vi "SpinningBooms.vi"() -> ()   [LabVIEW 2016]
doc: "The myRIO Project template acquires acceleration data from the onboard accelerometer and displays the changes of acceleration values in a waveform chart."
uses:
  <vilib>/myRIO/Common/Instrument Driver Framework/myRIO v1.0/Encoder/typedefs/Encoder Signal Mode.ctl
  <vilib>/myRIO/Instrument Drivers/Onboard IO/Encoder/typedefs/Encoder Reference.ctl
  <vilib>/myRIO/Common/Instrument Driver Framework/Utilities/typedefs/myRIO Generic Hardware Reference.ctl
  <vilib>/myRIO/Common/Instrument Driver Framework/Utilities/typedefs/Hardware Version Enum.ctl
  <vilib>/myRIO/Common/Instrument Driver Framework/Utilities/typedefs/myRIO v1.0 Reference.ctl
  <vilib>/myRIO/Common/Instrument Driver Framework/Utilities/typedefs/Generic FPGA Reference.ctl
  <vilib>/myRIO/Common/Instrument Driver Framework/myRIO v1.0/Encoder/typedefs/Encoder Channels Enum.ctl
  <vilib>/myRIO/Common/Instrument Driver Framework/myRIO v1.0/Encoder/typedefs/Encoder Configuration v1.0.ctl
  <vilib>/userdefined/High Color/nirio_resource_hc.ctl
  <vilib>/myRIO/Instrument Drivers/Onboard IO/PWM/typedefs/PWM Reference.ctl
  <vilib>/myRIO/Common/Instrument Driver Framework/myRIO v1.0/PWM/typedefs/PWM Channels Enum.ctl
  <vilib>/myRIO/Instrument Drivers/Onboard IO/PWM/typedefs/PWM Configuration.ctl
  <vilib>/myRIO/Common/Instrument Driver Framework/Utilities/vis/Is FPGA Ref Available.vi
  <vilib>/myRIO/Common/Instrument Driver Framework/myRIO v1.0/Encoder/vis/myRIO v1.1 Open Encoder.vi
  <vilib>/myRIO/Instrument Drivers/Onboard IO/Encoder/vis/Read.vi
  <vilib>/myRIO/Common/Instrument Driver Framework/myRIO v1.0/PWM/vis/myRIO v1.1 Open PWM.vi
  <vilib>/myRIO/Instrument Drivers/Onboard IO/PWM/vis/Set Duty Cycle and Frequency.vi
  <vilib>/myRIO/Common/Instrument Driver Framework/Utilities/vis/Validate Channels.vi
  <vilib>/myRIO/Common/Instrument Driver Framework/myRIO v1.0/Encoder/vis/myRIO v1.0 Reserve Encoder.vi
  <vilib>/myRIO/Common/Instrument Driver Framework/myRIO v1.0/PWM/vis/myRIO v1.0 Reserve PWM.vi
  <vilib>/myRIO/Common/Instrument Driver Framework/myRIO v1.0/UART/vis/myRIO v1.0 Close UART.vi
  <vilib>/myRIO/Common/Instrument Driver Framework/myRIO v1.0/Encoder/vis/myRIO v1.0 Build MUX Configuration Encoder.vi
  <vilib>/myRIO/Common/Instrument Driver Framework/myRIO v1.0/Resource Manager/vis/myRIO v1.0 Reserve Channel List.vi
  <vilib>/myRIO/Common/Instrument Driver Framework/myRIO v1.0/PWM/vis/myRIO v1.0 Build MUX Configuration PWM.vi
  <vilib>/myRIO/Common/Instrument Driver Framework/myRIO v1.0/Resource Manager/vis/myRIO v1.0 Create Configuration List.vi
  <vilib>/myRIO/Common/Instrument Driver Framework/myRIO v1.0/Resource Manager/vis/myRIO v1.0 Reserve Channel.vi
  <vilib>/myRIO/Common/Instrument Driver Framework/myRIO v1.0/Resource Manager/vis/myRIO v1.0 Unreserve Channel.vi
  <vilib>/myRIO/Common/Instrument Driver Framework/myRIO v1.0/Resource Manager/vis/myRIO v1.0 Build Mutex Name.vi
  <vilib>/Utility/VariantDataType/GetNumericInfo.vi
  <vilib>/Utility/error.llb/Error Cluster From Error Code.vi
  <vilib>/myRIO/Common/Instrument Driver Framework/myRIO v1.0/myRIO v1.1 Open.vi
  <vilib>/myRIO/Common/Instrument Driver Framework/Utilities/vis/IO Manager.vi
  <vilib>/myRIO/Common/Instrument Driver Framework/Utilities/vis/Configuration Manager.vi
  <vilib>/myRIO/Common/Instrument Driver Framework/myRIO v1.0/Resource Manager/vis/myRIO v1.0 Configure IO.vi
  <vilib>/myRIO/Common/Instrument Driver Framework/myRIO v1.0/myRIO v1.0 Close.vi
  <vilib>/myRIO/Common/Instrument Driver Framework/myRIO v1.0/Encoder/vis/myRIO v1.0 Configure Encoder.vi
  <vilib>/myRIO/Common/Instrument Driver Framework/myRIO v1.0/Encoder/vis/myRIO v1.0 Read Encoder.vi
  <vilib>/addons/control/pid/pid.llb/PID (DBL).vi
  <vilib>/myRIO/Common/Instrument Driver Framework/myRIO v1.0/PWM/vis/myRIO v1.0 Write PWM.vi
  <vilib>/myRIO/Common/Instrument Driver Framework/Utilities/vis/FPGA Ref Manager.vi
  <vilib>/myRIO/Common/Instrument Driver Framework/myRIO v1.0/myRIO v1.0 Reset FPGA.vi
  <vilib>/myRIO/Common/Instrument Driver Framework/myRIO v1.0/IRQ/vis/myRIO v1.0 IRQ Info FGV.vi
  <vilib>/myRIO/Common/Instrument Driver Framework/myRIO v1.0/IRQ/vis/myRIO v1.0 Timer IRQ Info FGV.vi
  <vilib>/myRIO/Common/Instrument Driver Framework/myRIO v1.0/IRQ/vis/myRIO v1.0 ISR Agent.vi
  <vilib>/myRIO/Express VI/Onboard IO/Encoder/Encoder Express VI.xnode
  <vilib>/myRIO/Instrument Drivers/Onboard IO/Encoder/vis/myRIO Encoder Open.xnode
  <vilib>/myRIO/Common/Instrument Driver Framework/myRIO v1.0/Encoder/typedefs/Encoder Count Direction Enum.ctl
  <vilib>/myRIO/Express VI/Onboard IO/PWM/PWM Express VI.xnode
  <vilib>/myRIO/Instrument Drivers/Onboard IO/PWM/vis/myRIO PWM Open.xnode
  <vilib>/myRIO/Instrument Drivers/Utilities/Utilities.lvlib
  <vilib>/myRIO/Instrument Drivers/Onboard IO/PWM/PWM.lvlib
  <vilib>/myRIO/Instrument Drivers/Onboard IO/Encoder/Encoder.lvlib
  <vilib>/addons/control/pid/NI_PID_pid.lvlib
panel:
  out "Rotations Per Minute 2":dbl(graph)
  out "Angular Velocity End 2":dbl(graph)
  out "rad/s 2":dbl
  out "Count Difference 2":dbl
  out "Angular Velocity 2":dbl(graph)
  out "Rotations Per Minute":dbl(graph)
  out "Rotations":dbl(graph)
  out "Rad End":dbl(graph)
  out "Angular Velocity End":dbl(graph)
  out "rad":dbl
  out "rad":dbl(graph)
  out "rad/s":dbl
  out "Count Difference":dbl
  out "Angular Velocity":dbl(graph)
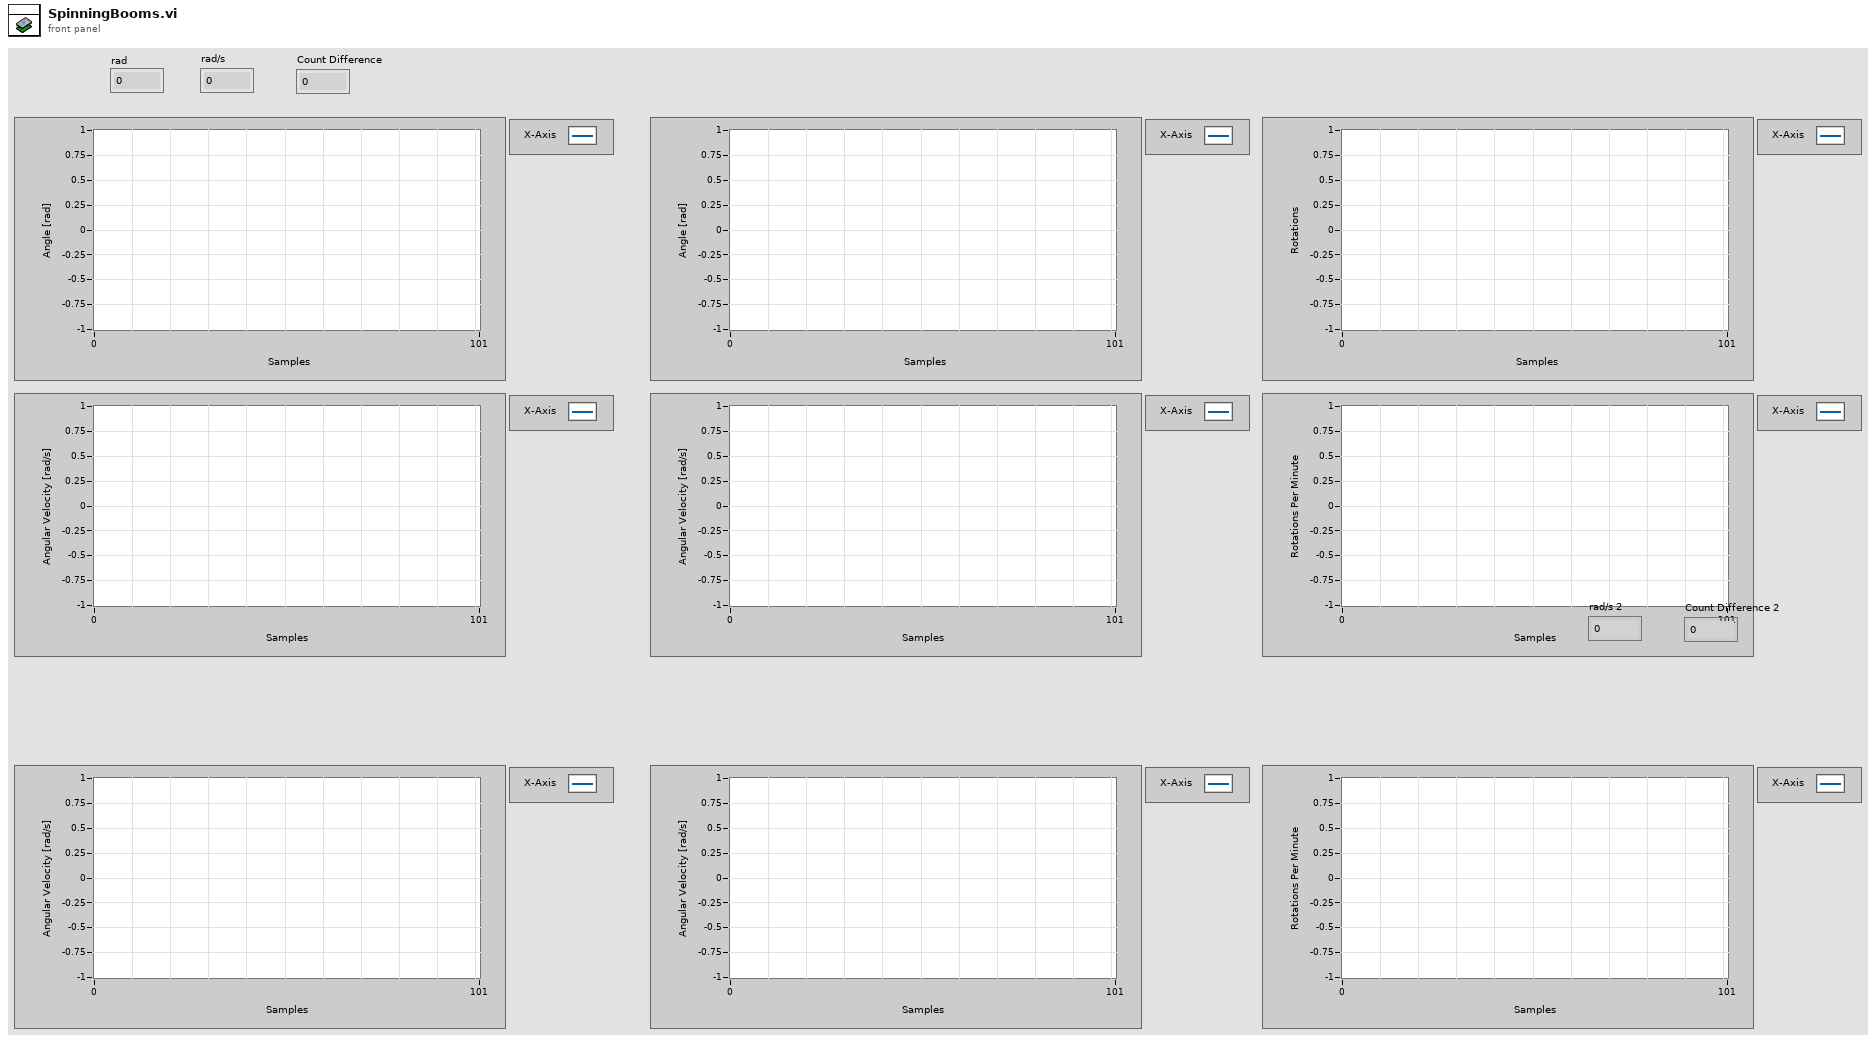
[diagram p1: front panel]
types:
  T1 = typedef "PWM.lvlib/PWM Reference.ctl" = cluster{"myRIO Reference":T2, "PWM Channels Enum":T6, "PWM Configuration":T7}
  T2 = typedef "myRIO Generic Hardware Reference.ctl" = cluster{"myRIO Model":T3, "myRIO Hardware Reference":T4}
  T3 = typedef "Hardware Version Enum.ctl" = enum16{"Unknown", "myRIO-1900", "myRIO-1950", "roboRIO", "NI ELVIS RIO CM"}
  T4 = typedef "myRIO v1.0 Reference.ctl" = cluster{"Generic FPGA Reference":T5, "Allow multiple opens":bool}
  T5 = typedef "Generic FPGA Reference.ctl" = refnum<k20>
  T6 = typedef "PWM Channels Enum.ctl" = enum16{"Not Connected", "C/PWM0", "C/PWM1", "A/PWM0", "A/PWM1", "A/PWM2", "B/PWM0", "B/PWM1", "B/PWM2", "PWM/PWM0", "PWM/PWM1", "PWM/PWM2", "PWM/PWM3", "PWM/PWM4", "PWM/PWM5", "PWM/PWM6", "PWM/PWM7", "PWM/PWM8", "PWM/PWM9"}
  T7 = typedef "PWM.lvlib/PWM Configuration.ctl" = cluster{"Frequency":dbl, "Duty Cycle":dbl}
  T8 = typedef "nirio_resource_hc.ctl" = tag
  T9 = typedef "Encoder.lvlib/Encoder Reference.ctl" = cluster{"myRIO Reference":T2, "Encoder Channels Enum":T10}
  T10 = typedef "Encoder Channels Enum.ctl" = enum16{"Not Connected", "C/ENC0", "C/ENC1", "A/ENC", "B/ENC", "DIO/ENC0", "DIO/ENC1", "DIO/ENC2", "DIO/ENC3", "DIO/ENC4"}
  T11 = typedef "Encoder Signal Mode.ctl" = enum16{"Quadrature phase signal", "Step and direction signal"}
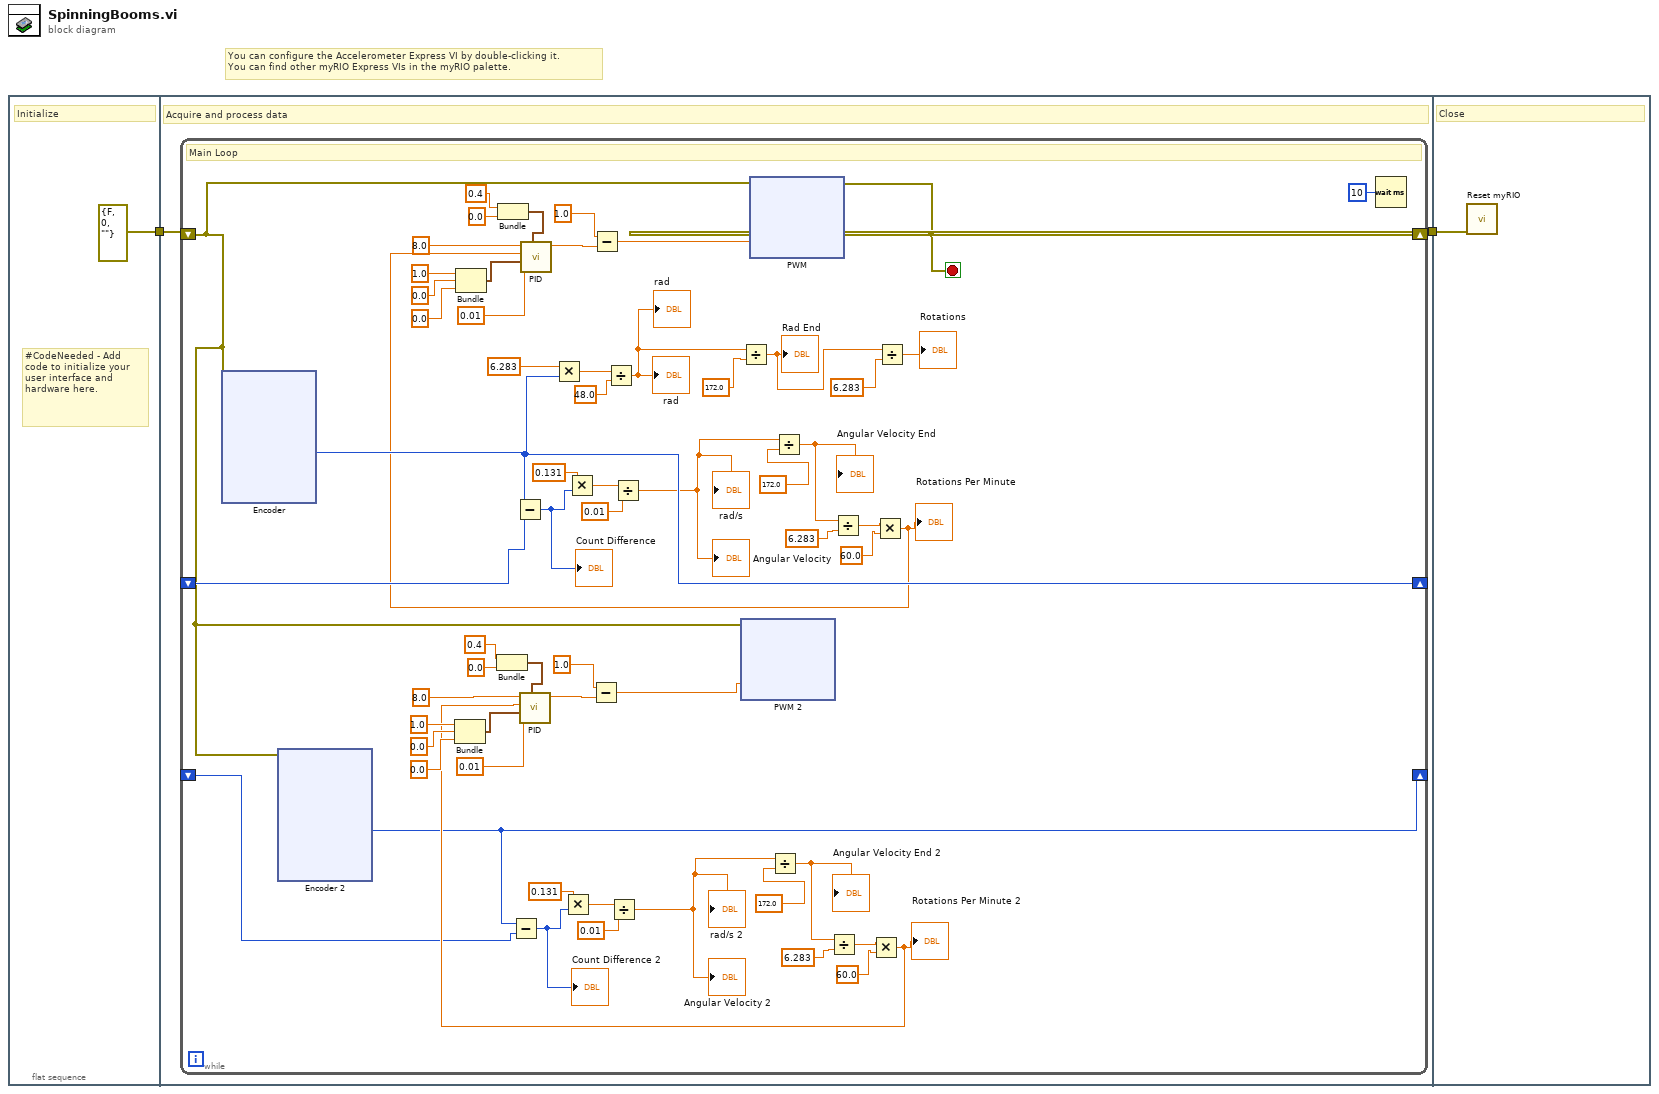
[diagram p0: block diagram]
diagram:
  # "You can configure the Accelerometer Express VI by double-clicking it.\nYou can find other myRIO Express VIs in the myRIO palette."
  n1 = flat-sequence {
    tunnel: [errorcluster {"status"=FALSE, "code"=0, "source"=""} ("error in (no error)")] -> w2
    tunnel: w2 -> [w5]
    tunnel: [w4] -> w1
    tunnel: w1 -> [w229]
    frame #0 {
      # "#CodeNeeded - Add code to initialize your user interface and hardware here."
      # "Initialize"
    }
    frame #1 {
      # "Acquire and process data"
      n2 = while {
        shift-right: [w56] -> w4
        shift-left: w5 -> [w33]
        shift-right: [w59] -> _
        shift-left: _ -> [w65]
        shift-right: [w7] -> _
        shift-left: _ -> [w6]
        stop <- w56 stop-if-true
        # "Main Loop"
        n3 = xnode "Encoder"("error in (no error)"=w33) -> ("Counter Value"=w59:i32)  [unwired: 1 in, 3 out]
        n4 = xnode "Encoder 2"("error in (no error)"=w33) -> ("Counter Value"=w7:i32)  [unwired: 1 in, 3 out]
        n5 = Bundle(1.0, 0.0, 0.0) -> (w27:cluster{dbl, dbl, dbl})  [unwired: 1 in]
        n6 = Bundle(1.0, 0.0, 0.0) -> (w38:cluster{dbl, dbl, dbl})  [unwired: 1 in]
        n7 = Bundle(0.4, 0.0) -> (w28:cluster{dbl, dbl})  [unwired: 1 in]
        n8 = Bundle(0.4, 0.0) -> (w40:cluster{dbl, dbl})  [unwired: 1 in]
        n9 = Subtract(x=w7, y=w6) -> (x-y=w15:i32)
        "Count Difference 2" <- w15
        n10 = Subtract(x=w59, y=w65) -> (x-y=w61:i32)
        "Count Difference" <- w61
        n11 = Multiply(x=6.283, y=w59) -> (x*y=w58:dbl)
        n12 = Multiply(x=0.131, y=w15) -> (x*y=w17:dbl)
        n13 = Multiply(x=0.131, y=w61) -> (x*y=w63:dbl)
        n14 = Divide(x=w58, y=48.0) -> (x/y=w55:dbl)
        "rad" <- w55
        "rad" <- w55
        n15 = Divide(x=w17, y=0.01) -> (x/y=w14:dbl)
        "Angular Velocity 2" <- w14
        "rad/s 2" <- w14
        n16 = Divide(x=w63, y=0.01) -> (x/y=w53:dbl)
        "Angular Velocity" <- w53
        "rad/s" <- w53
        n17 = Divide(x=w55, y=172.0) -> (x/y=w48:dbl)
        "Rad End" <- w48
        n18 = Divide(x=w14, y=172.0) -> (x/y=w12:dbl)
        "Angular Velocity End 2" <- w12
        n19 = Divide(x=w53, y=172.0) -> (x/y=w46:dbl)
        "Angular Velocity End" <- w46
        n20 = Divide(x=w12, y=6.283) -> (x/y=w10:dbl)
        n21 = Divide(x=w46, y=6.283) -> (x/y=w44:dbl)
        n22 = Multiply(x=w10, y=60.0) -> (x*y=w8:dbl)
        "Rotations Per Minute 2" <- w8
        n23 = call-poly <vilib>:"PID.vi"("output range"=w28, "dt (s)"=0.01, "PID gains"=w27, "process variable"=w8, "setpoint"=8.0) -> ("output"=w22:dbl)  [unwired: 5 in, 1 out]
        n24 = Subtract(x=1.0, y=w22) -> (x-y=w21:dbl)
        n25 = xnode "PWM 2"("Duty Cycle"=w21, "error in (no error)"=w33) -> ()  [unwired: 1 out]
        n26 = Multiply(x=w44, y=60.0) -> (x*y=w19:dbl)
        "Rotations Per Minute" <- w19
        n27 = call-poly <vilib>:"PID.vi"("output range"=w40, "dt (s)"=0.01, "PID gains"=w38, "process variable"=w19, "setpoint"=8.0) -> ("output"=w32:dbl)  [unwired: 5 in, 1 out]
        n28 = Subtract(x=1.0, y=w32) -> (x-y=w51:dbl)
        n29 = xnode "PWM"("Duty Cycle"=w51, "error in (no error)"=w33) -> ("error out"=w56:errorcluster)
        n30 = Divide(x=w48, y=6.283) -> (x/y=→"Rotations":dbl)
        n31 = Wait (ms)(milliseconds to wait=u32 10) -> ()  [unwired: 1 out]
      }
    }
    frame #2 {
      # "Close"
      n32 = call <vilib>:"Reset myRIO.vi"("error in (no error)"=w229) -> ()  [unwired: 10 in, 1 out]
    }
  }
